vi "Find tags bolds underline italic stikeoutVI.vi"(5 "Text":string, 11 "error in (no error)":errorcluster) -> (4 "Find tag ?":bool, 6 "Text out":string, 8 "Tags list [ ]":string[](array[string]), 10 "Tags position [ ]":i32[](array[numeric]), 15 "error out":errorcluster)   [LabVIEW 2019, in "Exaprom PDF.lvlib"]
doc: "Version 1.0\nDeveloped by Jean-Marc Simard\nCopyright © 2011, Exaprom Inc.\nAll rights reserved.\nLicense: BSD\n\nWith iTextSharp 4.1.6 (http://itextsharp.sourceforge.net)\nunder Mozilla Public License Version 1.1\n(http://www.mozilla.org/MPL/MPL-1.1.html)"
uses:
  Exaprom PDF.lvlib
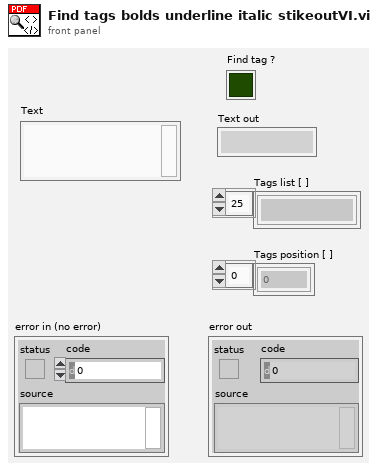
[diagram p1: front panel]
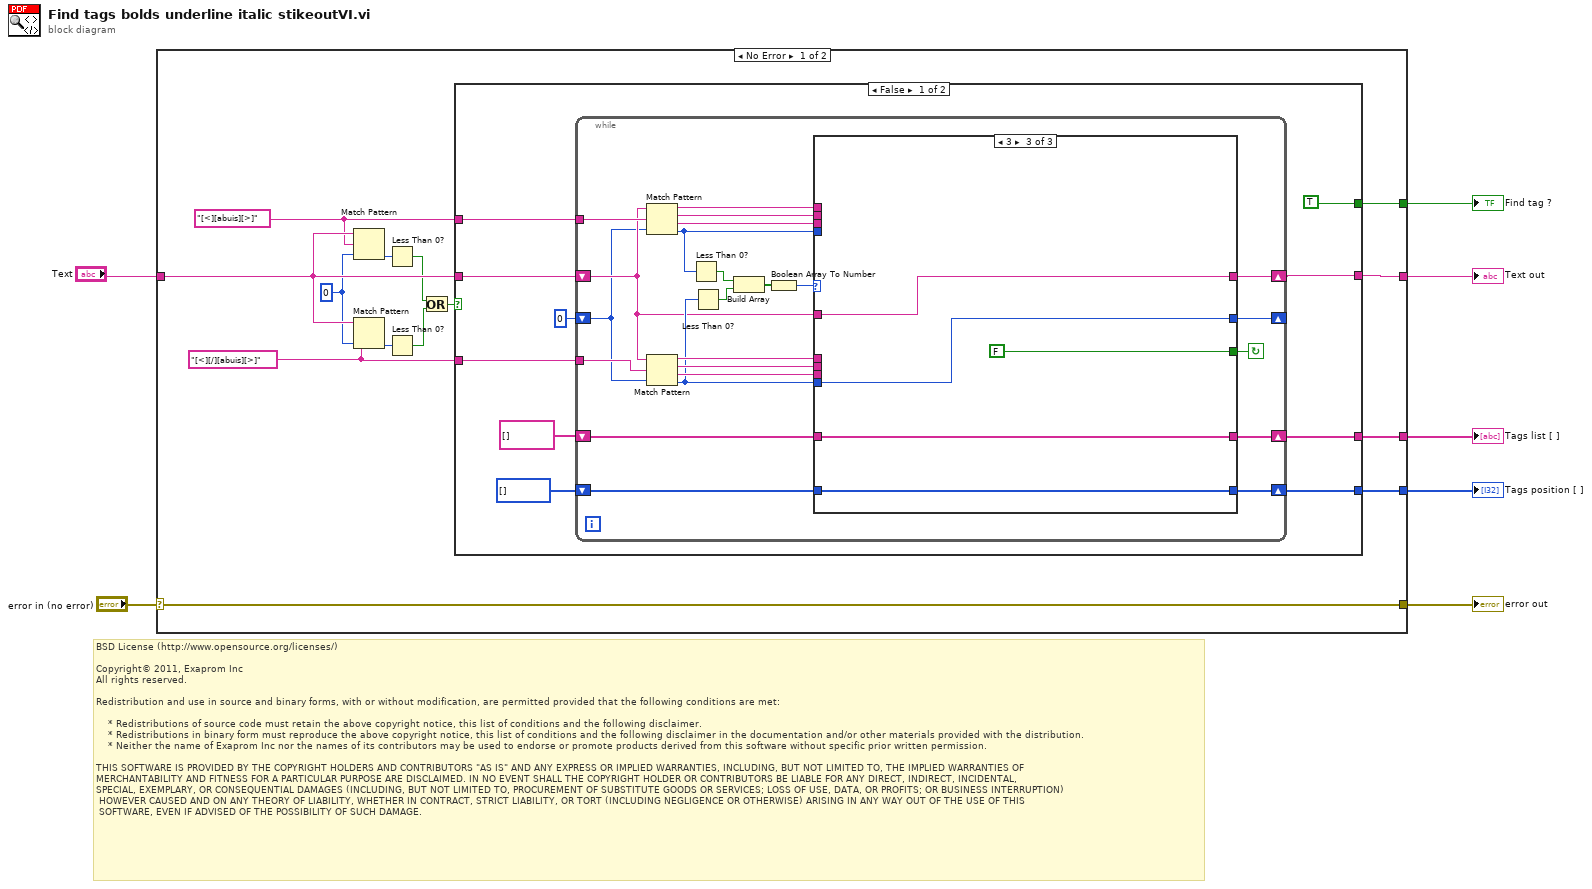
[diagram p0: block diagram]
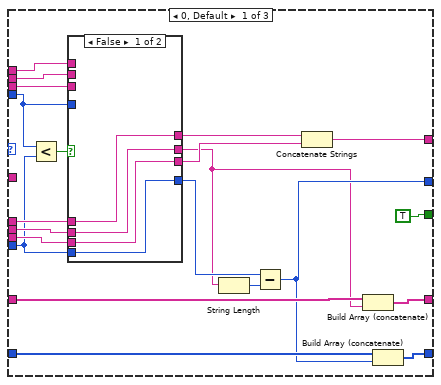
[diagram p2: hidden frame]
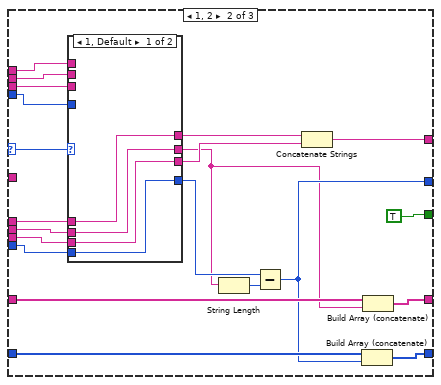
[diagram p4: hidden frame]
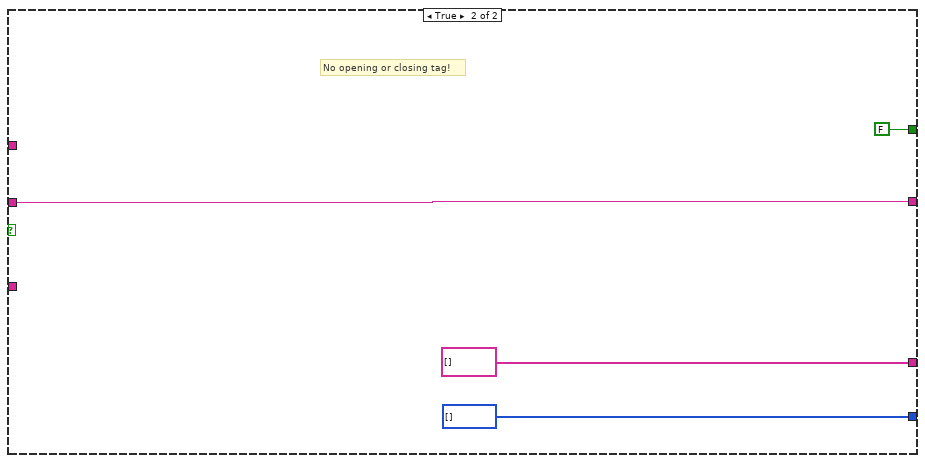
[diagram p6: hidden frame]
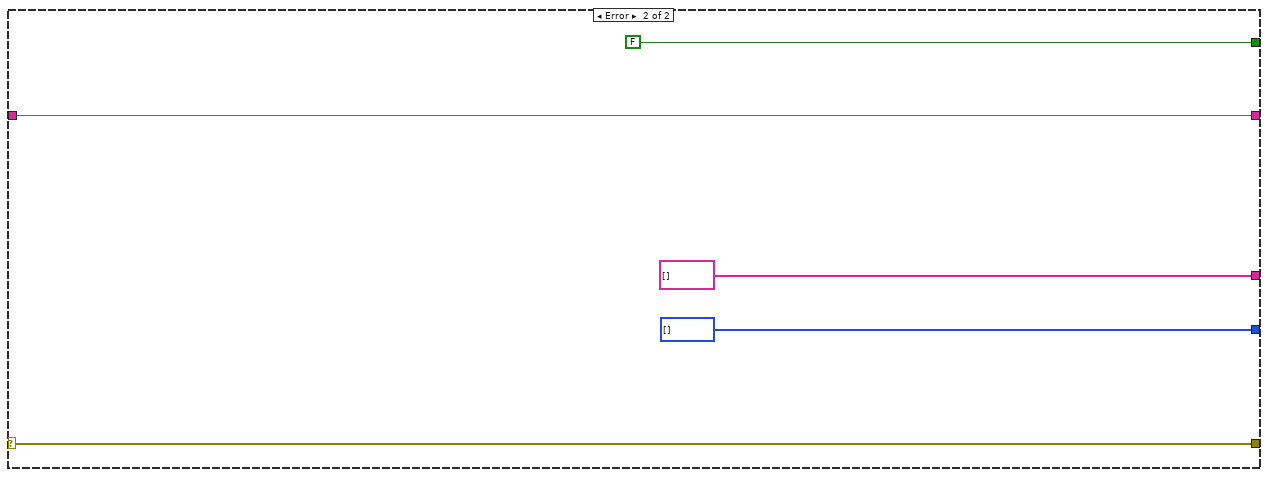
[diagram p7: hidden frame]
diagram:
  # "BSD License (http://www.opensource.org/licenses/)\n\nCopyright© 2011, Exaprom Inc\nAll rights reserved.\n\nRedistribution and use in source and binary forms, with or without modification, are permitted provided that the following conditions are met:\n\n    * Redistributions of source code must retain the above copyright notice, this list of conditions and the following disclaimer.\n    * Redistributions in binary form must reproduce the above copyright notice, this list of conditions and the following disclaimer in the documentation and/or other materials provided with the distribution.\n    * Neither the name of Exaprom Inc nor the names of its contributors may be used to endorse or promote products derived from this software without specific prior written permission.\n\nTHIS SOFTWARE IS PROVIDED BY THE COPYRIGHT HOLDERS AND CONTRIBUTORS \"AS IS\" AND ANY EXPRESS OR IMPLIED WARRANTIES, INCLUDING, BUT NOT LIMITED TO, THE IMPLIED WARRANTIES OF \nMERCHANTABILITY AND FITNESS FOR A PARTICULAR PURPOSE ARE DISCLAIMED. IN NO EVENT SHALL THE COPYRIGHT HOLDER OR CONTRIBUTORS BE LIABLE FOR ANY DIRECT, INDIRECT, INCIDENTAL,\nSPECIAL, EXEMPLARY, OR CONSEQUENTIAL DAMAGES (INCLUDING, BUT NOT LIMITED TO, PROCUREMENT OF SUBSTITUTE GOODS OR SERVICES; LOSS OF USE, DATA, OR PROFITS; OR BUSINESS INTERRUPTION)\n HOWEVER CAUSED AND ON ANY THEORY OF LIABILITY, WHETHER IN CONTRACT, STRICT LIABILITY, OR TORT (INCLUDING NEGLIGENCE OR OTHERWISE) ARISING IN ANY WAY OUT OF THE USE OF THIS\n SOFTWARE, EVEN IF ADVISED OF THE POSSIBILITY OF SUCH DAMAGE."
  n1 = case shown="No Error" "error in (no error)" {
    selector: "error in (no error)" -> [w21 w126]
    tunnel: [w21 w126] -> w7
    tunnel: "Text" -> [w20 w125]
    tunnel: [w11 w125] -> w4
    tunnel: [w10 string[] []] -> w3
    tunnel: [w9 i32[] []] -> w2
    tunnel: [w8 FALSE] -> w1
    frame No Error {
      w17 = 0
      w18 = "[<][/][abuis][>]"
      w19 = "[<][abuis][>]"
      n2 = Match Pattern(string=w20, regular expression=w19, offset (0)=w17) -> (offset past match=w15:i32)  [unwired: 3 out]
      n3 = Match Pattern(string=w20, regular expression=w18, offset (0)=w17) -> (offset past match=w16:i32)  [unwired: 3 out]
      n4 = Less Than 0?(x=w15) -> (x < 0?=w14:bool)
      n5 = Less Than 0?(x=w16) -> (x < 0?=w13:bool)
      n6 = Or(x=w14, y=w13) -> (x .or. y?=w12:bool)
      n7 = case shown="False" w12 {
        tunnel: w20 -> [w28 w121]
        tunnel: w19 -> [w27 _]
        tunnel: w18 -> [w26 _]
        tunnel: [w25 w121] -> w11
        tunnel: [w24 string[] []] -> w10
        tunnel: [w23 i32[] []] -> w9
        tunnel: [TRUE FALSE] -> w8
        frame False {
          n8 = while {
            tunnel: w26 -> [w54]
            shift-right: [w53] -> w24
            shift-left: string[] [] -> [w52]
            shift-right: [w44] -> _
            shift-left: 0 -> [w34]
            shift-right: [w47] -> w25
            shift-left: w28 -> [w43]
            tunnel: w27 -> [w46]
            shift-right: [w33] -> w23
            shift-left: i32[] [] -> [w32]
            stop <- w51 continue-if-true
            n9 = Match Pattern(string=w43, regular expression=w46, offset (0)=w34) -> (before substring=w38:string, match substring=w37:string, after substring=w36:string, offset past match=w35:i32)
            n10 = Match Pattern(string=w43, regular expression=w54, offset (0)=w34) -> (before substring=w48:string, match substring=w50:string, after substring=w49:string, offset past match=w45:i32)
            n11 = Less Than 0?(x=w35) -> (x < 0?=w42:bool)
            n12 = Less Than 0?(x=w45) -> (x < 0?=w41:bool)
            n13 = Build Array(w42, w41) -> (w40:bool[])
            n14 = Boolean Array To Number(Boolean array=w40) -> (number=w39:u32)
            n15 = case shown="3" w39 {
              selector: w39 -> [_ w88 _]
              tunnel: [w72 w101 w117] -> w53
              tunnel: w52 -> [w75 w104 w117]
              tunnel: [TRUE TRUE FALSE] -> w51
              tunnel: w50 -> [w68 w98 _]
              tunnel: w49 -> [w67 w97 _]
              tunnel: w48 -> [w69 w99 _]
              tunnel: [w73 w102 w114] -> w47
              tunnel: w45 -> [w66 w96 w115]
              tunnel: [w56 w86 w115] -> w44
              tunnel: w43 -> [_ _ w114]
              tunnel: w38 -> [w62 w92 _]
              tunnel: w37 -> [w61 w91 _]
              tunnel: w36 -> [w60 w90 _]
              tunnel: w35 -> [w59 w89 _]
              tunnel: [w58 w85 w113] -> w33
              tunnel: w32 -> [w57 w87 w113]
              frame 0, Default {
                n16 = Less?(x=w59, y=w66) -> (x < y?=w70:bool)
                n17 = case shown="False" w70 {
                  tunnel: [w79 w83] -> w63
                  tunnel: w69 -> [w79 _]
                  tunnel: [w78 w82] -> w55
                  tunnel: w68 -> [w78 _]
                  tunnel: [w77 w81] -> w64
                  tunnel: w67 -> [w77 _]
                  tunnel: [w76 w80] -> w65
                  tunnel: w66 -> [w76 _]
                  tunnel: w62 -> [_ w83]
                  tunnel: w61 -> [_ w82]
                  tunnel: w60 -> [_ w81]
                  tunnel: w59 -> [_ w80]
                  frame False {
                  }
                  frame True {
                  }
                }
                n18 = String Length(string=w55) -> (length=w74:i32)
                n19 = Subtract(x=w65, y=w74) -> (x-y=w56:i32)
                n20 = Concatenate Strings(w63, w64) -> (w73:string)
                n21 = Build Array (concatenate)(w75, w55) -> (w72:string[])
                n22 = Build Array (concatenate)(w57, w56) -> (w58:i32[])
              }
              frame 1, 2 {
                n23 = case shown="1, Default" w88 {
                  tunnel: [w108 w112] -> w93
                  tunnel: w99 -> [w108 _]
                  tunnel: [w107 w111] -> w84
                  tunnel: w98 -> [w107 _]
                  tunnel: [w106 w110] -> w94
                  tunnel: w97 -> [w106 _]
                  tunnel: [w105 w109] -> w95
                  tunnel: w96 -> [w105 _]
                  tunnel: w92 -> [_ w112]
                  tunnel: w91 -> [_ w111]
                  tunnel: w90 -> [_ w110]
                  tunnel: w89 -> [_ w109]
                  frame 1, Default {
                  }
                  frame 2 {
                  }
                }
                n24 = String Length(string=w84) -> (length=w103:i32)
                n25 = Subtract(x=w95, y=w103) -> (x-y=w86:i32)
                n26 = Concatenate Strings(w93, w94) -> (w102:string)
                n27 = Build Array (concatenate)(w87, w86) -> (w85:i32[])
                n28 = Build Array (concatenate)(w104, w84) -> (w101:string[])
              }
              frame 3 {
              }
            }
          }
        }
        frame True {
          # "No opening or closing tag!"
        }
      }
    }
    frame Error {
    }
  }
  "error out" <- w7
  "Text out" <- w4
  "Tags list [ ]" <- w3
  "Tags position [ ]" <- w2
  "Find tag ?" <- w1
